vi "Initialize UI.vi"(8 "error in (no error)":errorcluster, 11 "Application in":refnum<class "Application.lvclass">) -> (0 "error out":errorcluster, 3 "Application out":refnum<class "Application.lvclass">)   [LabVIEW 2023, in "Application.lvlib" / "Application.lvclass"]
uses:
  Application.lvclass
  C:/Program Files/National Instruments/LabVIEW 2023/vi.lib/ActorFramework/Actor/Actor.lvclass
  Services/Particle Counter/Particle Counter/Particle Counter.lvclass
  Application.lvclass/Application.ctl
  User Interface/Splash Screen Messages/Update Status Msg/Update Status Msg.lvclass/Update Status Msg.ctl
  <vilib>/ActorFramework/Message Enqueuer/Message Enqueuer.lvclass/Message Enqueuer.ctl
  <vilib>/ActorFramework/Message Enqueuer/Enqueue.vi
  User Interface/Splash Screen Messages/Update Status Msg/Update Status Msg.lvclass
  C:/Program Files/National Instruments/LabVIEW 2023/vi.lib/ActorFramework/Message/Message.lvclass
  <vilib>/ActorFramework/Message Priority Queue/Priority Enqueue.vi
  <vilib>/ActorFramework/Actor/Actor.lvclass
  Automation/AutomationContext.lvclass
  C:/FlashGordon/Development/Application/Application.lvclass
  C:/FlashGordon/Development/Services/Particle Counter/Particle Counter/Particle Counter.lvclass
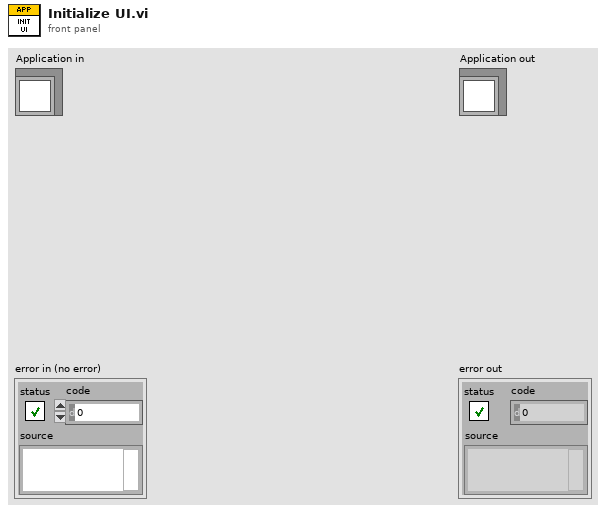
[diagram p1: front panel]
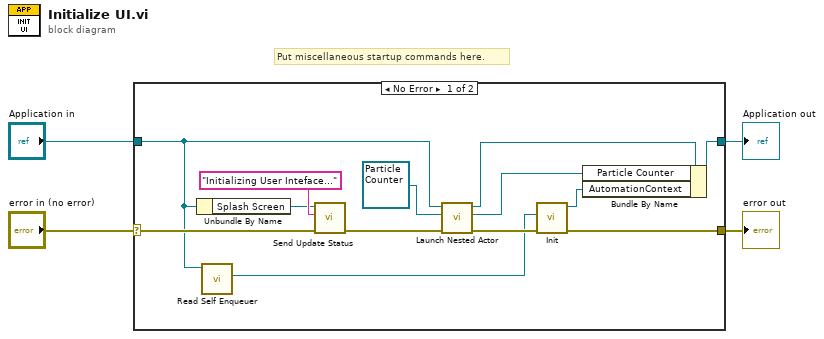
[diagram p0: block diagram]
diagram:
  # "Put miscellaneous startup commands here."
  n1 = case shown="No Error" "error in (no error)" {
    selector: "error in (no error)" -> [w15 w19]
    tunnel: [w8 w19] -> w3
    tunnel: [w14 w18] -> w1
    tunnel: "Application in" -> [w6 w18]
    frame No Error {
      n2 = Unbundle By Name(w6) -> ("Splash Screen"=w16:refnum<class "Message Enqueuer.lvclass">)
      n3 = call <vilib>:"Read Self Enqueuer.vi"("Actor"=w6) -> ("Self Enqueuer"=w5:refnum<class "Message Enqueuer.lvclass">)  [unwired: 10 in]
      n4 = call "Send Update Status.vi"("error in (no error)"=w15, "Status Message"="Initializing User Inteface...", "Message Enqueuer"=w16) -> ("error out"=w13:errorcluster)  [unwired: 7 in, 1 out]
      n5 = call <vilib>:"Launch Nested Actor.vi"("error in (no error)"=w13, "Nested Actor"=refnum<class "Particle Counter.lvclass"> refnum ("Particle Counter.lvlib:Particle Counter.lvclass"), "Caller Actor in"=w6) -> ("error out"=w9:errorcluster, "Nested Actor's Enqueuer"=w12:refnum<class "Message Enqueuer.lvclass">, "Caller Actor out"=w11:refnum<class "Application.lvclass">)  [unwired: 6 in]
      n6 = call "Init.vi"("error in (no error)"=w9, "Application Ref"=w5) -> ("error out"=w8:errorcluster, "AutomationContext out"=w7:refnum<class "AutomationContext.lvclass">)  [unwired: 8 in]
      n7 = Bundle By Name(cluster=w11, "Particle Counter"=w12, "AutomationContext"=w7) -> (w14:refnum<class "Application.lvclass">)
    }
    frame Error {
    }
  }
  "error out" <- w3
  "Application out" <- w1
